vi "InitialiseAttributesAndMethods.vi"(8 "error in (no error)":errorcluster, 11 "ParseMermaid in":refnum<class "ParseMermaid.lvclass">) -> (0 "error out":errorcluster, 3 "ParseMermaid out":refnum<class "ParseMermaid.lvclass">)   [LabVIEW 2020, in "Mermaid.lvlib" / "ParseMermaid.lvclass"]
uses:
  ParseMermaid.lvclass
  ParseMermaid.lvclass/ParseMermaid.ctl
  <vilib>/regexp/Match Regular Expression.xnode
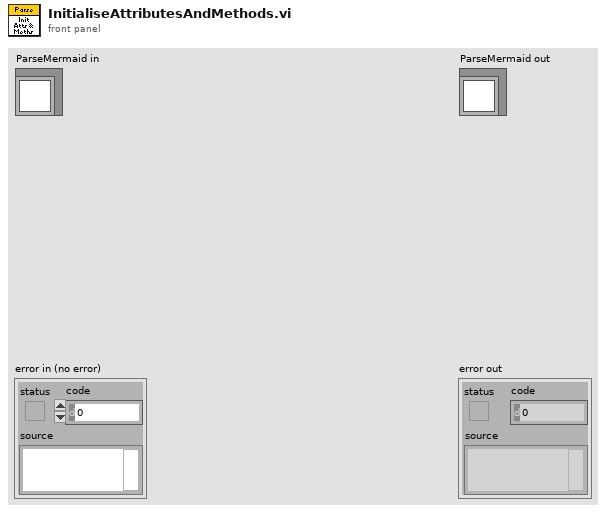
[diagram p1: front panel]
types:
  T1 = typedef "Mermaid.lvlib/ParseMermaid.lvclass/ClassData.ctl" = cluster{"Name":string, "ClassType":T2, "PublicMethods":string[], "PrivateMethods":string[], "FinalPublicAttributes":T3, "FinalPrivateAttributes":T3, "Parent":string}
  T2 = typedef "Mermaid.lvlib/ParseMermaid.lvclass/ClassType.ctl" = enum16{"Interface", "Class"}
  T3 = typedef "Mermaid.lvlib/ParseMermaid.lvclass/Attributes.ctl" = cluster{"Name":string, "Type":i32}[]
  T4 = typedef "Mermaid.lvlib/ParseMermaid.lvclass/Attribute.ctl" = cluster{"Name":string, "Type":i32}
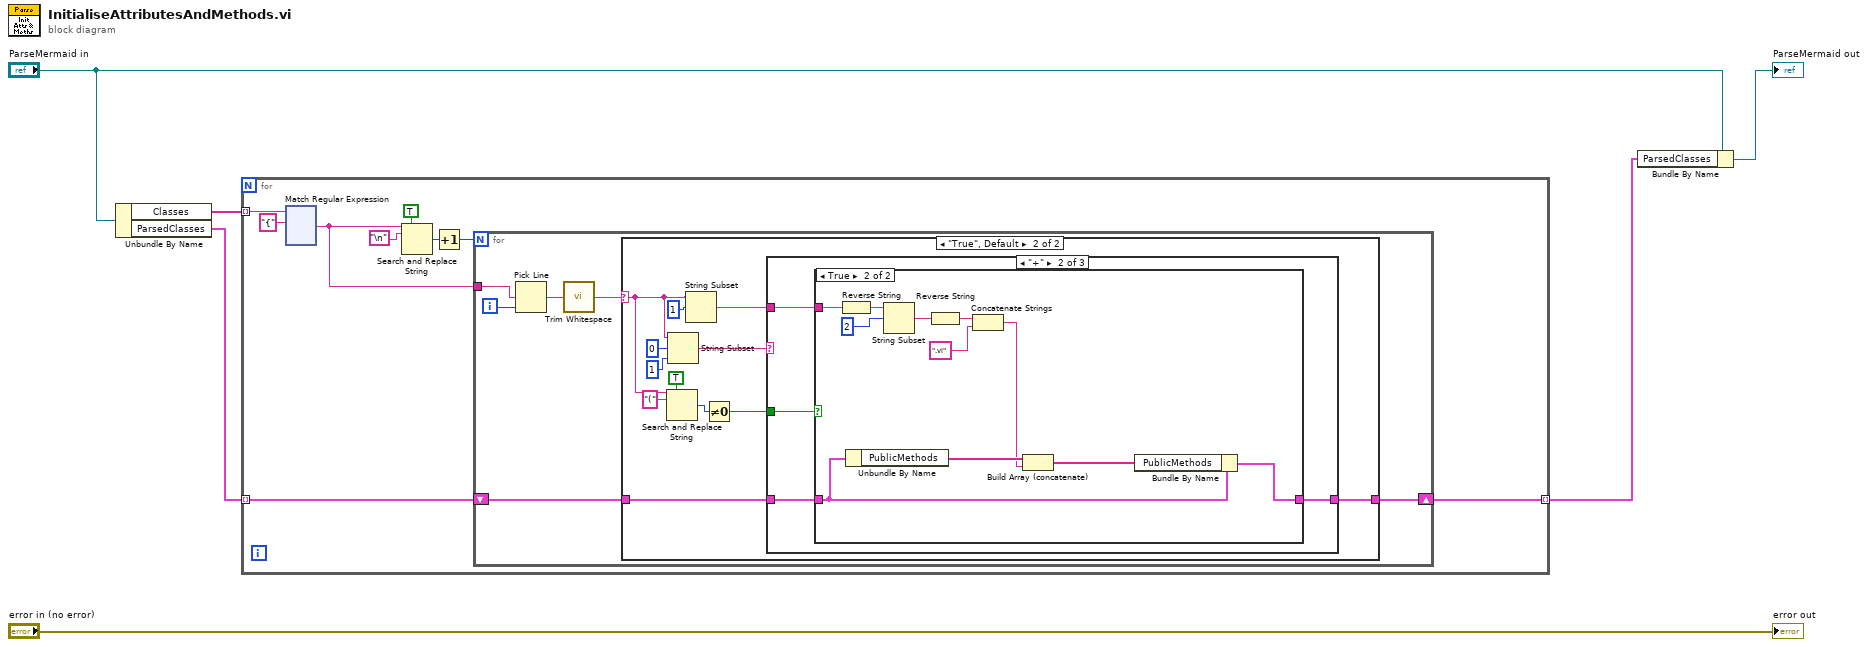
[diagram p0: block diagram]
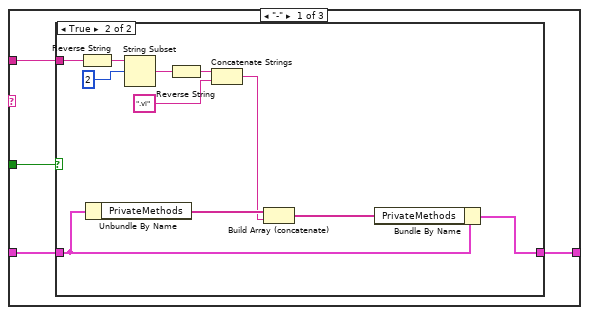
[diagram p3: hidden frame]
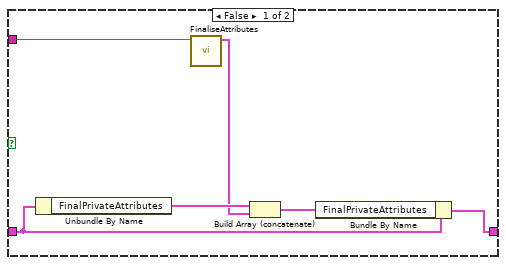
[diagram p4: hidden frame]
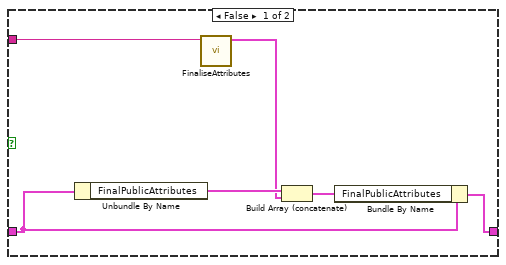
[diagram p5: hidden frame]
diagram:
  n1 = Unbundle By Name("ParseMermaid in") -> ("Classes"=w5:string[], "ParsedClasses"=w4:T1[])
  n2 = for {
    tunnel: w4 -> [w10] mode=indexing
    tunnel: w5 -> [w14] mode=indexing
    tunnel: [w9] -> w3 mode=indexing
    n3 = xnode "Match Regular Expression"("input string"=w14, "regular expression"="{") -> ("after match"=w7:string)  [unwired: 4 in, 4 out]
    n4 = Search and Replace String(replace all?=TRUE ("replace all? (F)"), input string=w7, search string="\n") -> (number of replacements=w13:i32)  [unwired: 5 in, 3 out]
    n5 = Increment(x=w13) -> (x+1=w8:i32)
    n6 = for {
      N: w8 -> [_]
      shift-right: [w19] -> w9
      shift-left: w10 -> [w20]
      tunnel: w7 -> [w18]
      i -> [w21]
      n7 = Pick Line(multi-line string=w18, line index=w21) -> (output string=w17:string)  [unwired: 1 in]
      n8 = call <vilib>:"Trim Whitespace.vi"("string"=w17) -> ("trimmed string"=w16:string)  [unwired: 1 in]
      n9 = case shown="\"True\", Default" w16 {
        selector: w16 -> [_ w28]
        tunnel: w20 -> [w22 w25]
        tunnel: [w22 w24] -> w19
        frame "" {
        }
        frame "True", Default {
          n10 = Search and Replace String(replace all?=TRUE ("replace all? (F)"), input string=w28, search string="(") -> (number of replacements=w23:i32)  [unwired: 5 in, 3 out]
          n11 = String Subset(string=w28, offset (0)=0, length (rest)=1 ("length (rest)")) -> (substring=w32:string)
          n12 = String Subset(string=w28, offset (0)=1) -> (substring=w26:string)  [unwired: 1 in]
          n13 = Not Equal To 0?(x=w23) -> (x != 0?=w29:bool)
          n14 = case shown="\"+\"" w32 {
            tunnel: w29 -> [w37 w59 _]
            tunnel: w26 -> [w36 w57 _]
            tunnel: w25 -> [w38 w58 w77]
            tunnel: [w35 w56 w77] -> w24
            frame "-" {
              n15 = case shown="True" w37 {
                tunnel: w38 -> [w44 w50]
                tunnel: w36 -> [w40 w55]
                tunnel: [w41 w48] -> w35
                frame False {
                  n16 = Unbundle By Name(w44) -> ("FinalPrivateAttributes"=w43:T3)
                  n17 = call "FinaliseAttributes.vi"("String"=w40) -> ("output cluster"=w39:T4)  [unwired: 10 in]
                  n18 = Build Array (concatenate)(w43, w39) -> (w42:T4[])
                  n19 = Bundle By Name(cluster=w44, "FinalPrivateAttributes"=w42) -> (w41:T1)
                }
                frame True {
                  n20 = Reverse String(1:w55) -> (0:w54:string)
                  n21 = Unbundle By Name(w50) -> ("PrivateMethods"=w51:string[])
                  n22 = String Subset(string=w54, offset (0)=2) -> (substring=w52:string)  [unwired: 1 in]
                  n23 = Reverse String(1:w52) -> (0:w47:string)
                  n24 = Concatenate Strings(w47, ".vi" ("string")) -> (w45:string)
                  n25 = Build Array (concatenate)(w51, w45) -> (w49:string[])
                  n26 = Bundle By Name(cluster=w50, "PrivateMethods"=w49) -> (w48:T1)
                }
              }
            }
            frame "+" {
              n27 = case shown="True" w59 {
                tunnel: w58 -> [w64 w71]
                tunnel: w57 -> [w61 w76]
                tunnel: [w62 w69] -> w56
                frame False {
                  n28 = Unbundle By Name(w64) -> ("FinalPublicAttributes"=w65:T3)
                  n29 = call "FinaliseAttributes.vi"("String"=w61) -> ("output cluster"=w60:T4)  [unwired: 10 in]
                  n30 = Build Array (concatenate)(w65, w60) -> (w63:T4[])
                  n31 = Bundle By Name(cluster=w64, "FinalPublicAttributes"=w63) -> (w62:T1)
                }
                frame True {
                  n32 = Reverse String(1:w76) -> (0:w75:string)
                  n33 = Unbundle By Name(w71) -> ("PublicMethods"=w72:string[])
                  n34 = String Subset(string=w75, offset (0)=2) -> (substring=w73:string)  [unwired: 1 in]
                  n35 = Reverse String(1:w73) -> (0:w68:string)
                  n36 = Concatenate Strings(w68, ".vi" ("string")) -> (w67:string)
                  n37 = Build Array (concatenate)(w72, w67) -> (w70:string[])
                  n38 = Bundle By Name(cluster=w71, "PublicMethods"=w70) -> (w69:T1)
                }
              }
            }
            frame Default {
              # "Some terrible error"
            }
          }
        }
      }
    }
  }
  n39 = Bundle By Name(cluster="ParseMermaid in", "ParsedClasses"=w3) -> (→"ParseMermaid out":refnum<class "ParseMermaid.lvclass">)
  "error out" <- "error in (no error)"
